vi "Clean Up Block Diagram.vi"(6 "VI Path":path, 8 "error in (no error)":errorcluster) -> (0 "error out":errorcluster)   [LabVIEW 2017]
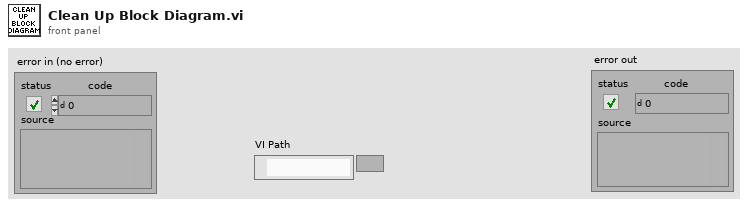
[diagram p1: front panel]
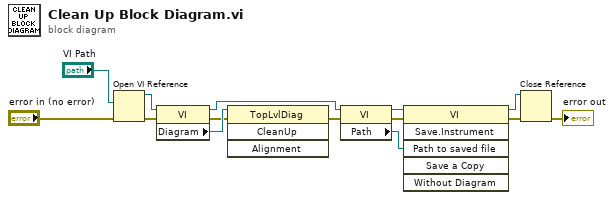
[diagram p0: block diagram]
diagram:
  n1 = Open VI Reference(vi path="VI Path", error in (no error)="error in (no error)") -> (vi reference=w14:refnum<vi>, error out=w13:errorcluster)  [unwired: 4 in]
  n2 = property class="VI"(reference=w14, error in=w13) -> (reference out=w4:refnum<vi>, error out=w11:errorcluster, "Diagram"=w12:refnum<vi>)
  n3 = invoke class="TopLvlDiag" method="CleanUp"(reference=w12, error in=w11) -> (error out=w9:errorcluster)  [unwired: 2 in, 3 out]
  n4 = property class="VI"(reference=w4, error in=w9) -> (reference out=w3:refnum<vi>, error out=w5:errorcluster, "Path"=w2:path)
  n5 = invoke class="VI" method="Save.Instrument"(reference=w3, error in=w5, "Path to saved file"=w2) -> (reference out=w1:refnum<vi>, error out=w7:errorcluster)  [unwired: 3 in, 4 out]
  n6 = Close Reference(reference=w1, error in (no error)=w7) -> (error out=→"error out":errorcluster)
